vi "PCO_Grab_Save.vi"(7 "# of frames":u16, 8 "entrée d'erreur (pas d'erreur)":errorcluster, 9 "Message Data":variant, 10 "notifier out":refnum<notifier>, 11 "Camera en entrée":refnum<class "Camera.lvclass">) -> (0 "sortie d'erreur":errorcluster, 2 "Raw data (U16)":u16[][][](array[numeric]), 3 "Camera en sortie":refnum<class "Camera.lvclass">)   [LabVIEW 2026]
uses:
  pco.labview/camera/Camera.lvclass
  Controls/PCO_Config.ctl
panel:
  out "recorded_image_count":u32
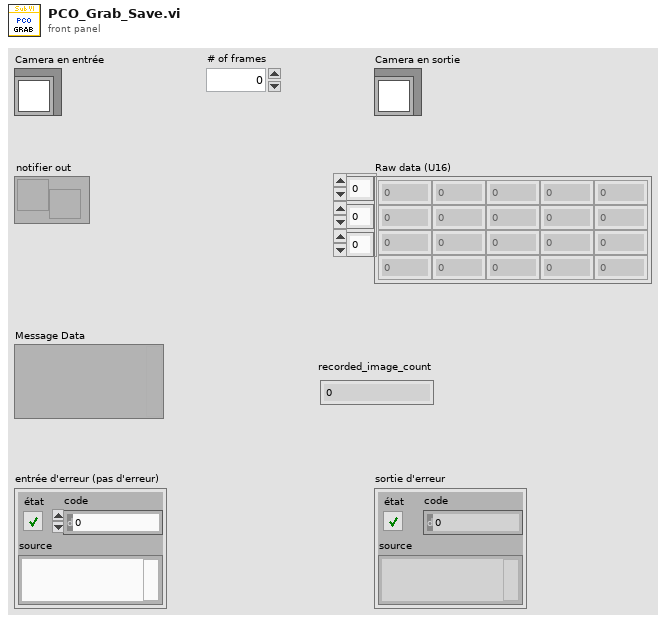
[diagram p1: front panel]
types:
  T1 = enum16{"sequence", "sequence non blocking", "ring buffer", "fifo", "tif", "multitif", "pcoraw", "b16", "dicom", "multidicom", "camram_ring", "camram_segment"}
  T2 = enum16{"Undefined", "Mono8", "Mono16", "BGRA8", "RGBA8", "BGRA16", "RGBA16", "CompressedMono8"}
  T3 = typedef "PCO_Config.ctl" = cluster{"Exposure time (s)":dbl, "TriggerMode":u16, "ROI X0":u16, "ROI Y0":u16, "ROI X1":u16, "ROI Y1":u16, "Binning":u8}
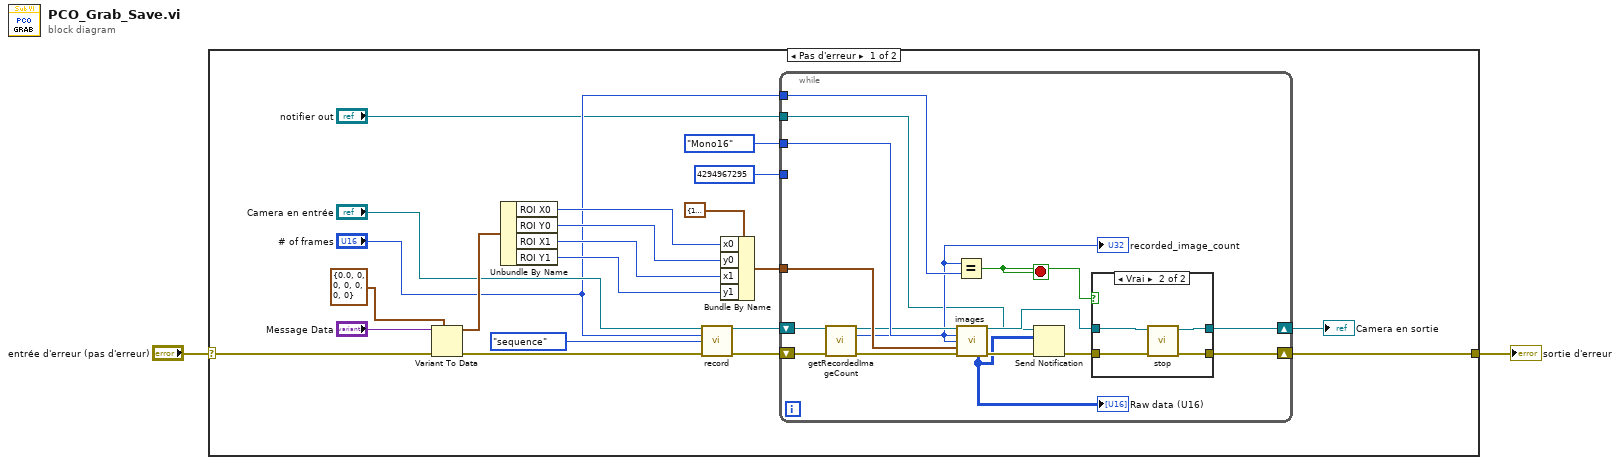
[diagram p0: block diagram]
diagram:
  n1 = case shown="Pas d'erreur" "entrée d'erreur (pas d'erreur)" {
    selector: "entrée d'erreur (pas d'erreur)" -> [w8 w46]
    tunnel: [w7 w46] -> w2
    frame No Error {
      n2 = Variant To Data(error in=w8, type=T3 {"Exposure time (s)"=0.0, "TriggerMode"=0, "ROI X0"=0, "ROI Y0"=0, "ROI X1"=0, "ROI Y1"=0, "Binning"=0} ("PCO_Config"), Variant="Message Data") -> (data=w17:T3, error out=w14:errorcluster)
      n3 = Unbundle By Name(w17) -> ("ROI X0"=w21:u16, "ROI Y0"=w20:u16, "ROI X1"=w19:u16, "ROI Y1"=w18:u16)
      n4 = call-dynamic "record.vi"("Camera in"="Camera en entrée", "num_images"="# of frames", "record_mode"=T1."sequence", "error in (no error)"=w14) -> ("Camera out"=w9:refnum<class "Camera.lvclass">, "error out"=w10:errorcluster)  [unwired: 10 in]
      n5 = Bundle By Name(cluster=cluster{"x0":u64, "y0":u64, "x1":u64, "y1":u64} {"x0"=18446744073709551615, "y0"=18446744073709551615, "x1"=18446744073709551615, "y1"=18446744073709551615} ("roi"), "x0"=w21, "y0"=w20, "x1"=w19, "y1"=w18) -> (w22:cluster{"x0":u64, "y0":u64, "x1":u64, "y1":u64})
      n6 = while {
        tunnel: T2."Mono16" ("data_format") -> [w39]
        tunnel: w22 -> [w38]
        tunnel: u32 4294967295 ("dwImgIdx") -> [_]
        shift-right: [w24] -> w7
        shift-left: w10 -> [w35]
        shift-right: [w31] -> w11
        shift-left: w9 -> [w34]
        tunnel: "# of frames" -> [w33]
        tunnel: "notifier out" -> [w27]
        stop <- w30 stop-if-true
        n7 = call-dynamic "getRecordedImageCount.vi"("Camera in"=w34, "error in (no error)"=w35) -> ("Camera out"=w36:refnum<class "Camera.lvclass">, "recorded_image_count"=w29:u32, "error out"=w37:errorcluster)  [unwired: 11 in]
        "recorded_image_count" <- w29
        n8 = Equal?(x=w29, y=w33) -> (x = y?=w30:bool)
        n9 = call-dynamic "images.vi"("Camera in"=w36, "data_format"=w39, "image_count"=w29, "crop"=w38, "error in (no error)"=w37) -> ("Camera out"=w32:refnum<class "Camera.lvclass">, "raw_image_list (U16)"=w25:u16[][][], "error out"=w28:errorcluster)  [unwired: 2 in, 6 out]
        "Raw data (U16)" <- w25
        n10 = Send Notification(notification=w25, notifier=w27, error in (no error)=w28) -> (error out=w26:errorcluster)  [unwired: 1 out]
        n11 = case shown="Vrai" w30 {
          tunnel: w26 -> [w41 w45]
          tunnel: [w41 w44] -> w24
          tunnel: w32 -> [w40 w43]
          tunnel: [w40 w42] -> w31
          frame False {
          }
          frame True {
            n12 = call-dynamic "stop.vi"("error in (no error)"=w45, "Camera in"=w43) -> ("error out"=w44:errorcluster, "Camera out"=w42:refnum<class "Camera.lvclass">)  [unwired: 8 in]
          }
        }
      }
      "Camera en sortie" <- w11
    }
    frame Error {
    }
  }
  "sortie d'erreur" <- w2
